vi "GSM Configure Hardware.vi"(0 "VISA Resource Name":refnum<visa-resource-name>, 7 "External 13 MHz (F:OFF)":bool, 9 "BBG Data Clock (F:INT)":bool, 11 "error in (no error)":errorcluster {"code" format="%.0x"}) -> (4 "VISA Resource Name Out":refnum<visa-resource-name>, 15 "error out":errorcluster {"code" format="%.0x"})   [LabVIEW 2012, in "Agilent ESG Series.lvlib"]
doc: "This VI is used to configure the \"Configure Hardware\" parameters."
uses:
  <instrlib>/Agilent ESG Series/Agilent ESG Series.lvlib
panel:
  # "ON"
  # "OFF"
  # "EXT"
  # "INT"
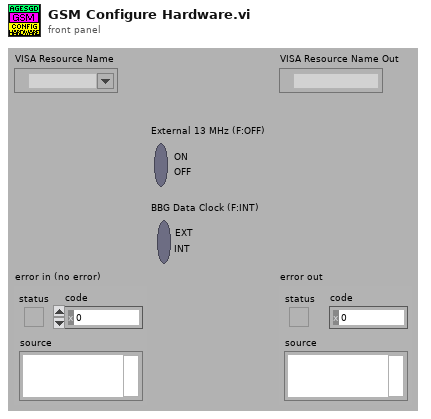
[diagram p1: front panel]
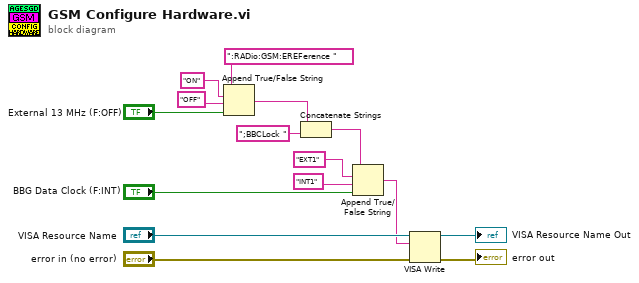
[diagram p0: block diagram]
diagram:
  n1 = Append True/False String(1:"External 13 MHz (F:OFF)", 2:"OFF" ("false string"), 3:"ON" ("true string"), 4:":RADio:GSM:EREFerence ") -> (0:w3:string)
  n2 = Concatenate Strings(w3, ";BBCLock ") -> (w4:string)
  n3 = Append True/False String(1:"BBG Data Clock (F:INT)", 2:"INT1" ("false string"), 3:"EXT1" ("true string"), 4:w4) -> (0:w1:string)
  n4 = VISA Write(VISA resource name="VISA Resource Name", write buffer=w1, error in (no error)="error in (no error)") -> (VISA resource name out=→"VISA Resource Name Out":refnum<visa-resource-name>, error out=→"error out":errorcluster)  [unwired: 1 out]
